vi "NanotecSMCPD.get parameters.vi"(0 "i ref in":refnum<vi>, 5 "error in (no error)":errorcluster) -> (7 "ReverseDirection?":bool[](array[boolean]), 8 "startFrequency [unit/s]":dbl[](array[numeric]), 9 "PhaseCurrent [A]":dbl[](array[numeric]), 11 "name":string[](array[string]), 12 "stopFrequency [unit/s]":dbl[](array[numeric]), 13 "unit":string[](array[string]), 14 "i ref out":refnum<vi>, 15 "acceleration [unit/s^2]":dbl[](array[numeric]), 16 "minRange [unit]":dbl[](array[numeric]), 17 "maxRange[unit]":dbl[](array[numeric]), 18 "scaling [unit]":dbl[](array[numeric]), 19 "error out":errorcluster)   [LabVIEW 2014, in "NanotecSMCPD.lvlib"]
doc: "Gets the parameters required for configuring the axes."
uses:
  NanotecSMCPD.lvlib
  CS_Core/BaseProcess/BaseProcess.lvlib
  CS_Core/CSSystem/CoreLib/CoreLib.lvlib
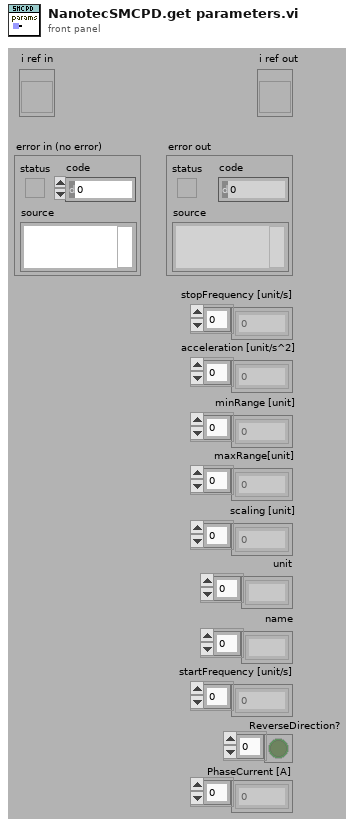
[diagram p1: front panel]
types:
  T1 = typedef "BaseProcess.lvlib/BaseProcess.i attribute.ctl" = cluster{"EventStatus":string, "EventError":i32, "PresetEvtWatchD":i32, "PresetPdcWatchD":i32, "EventTimeout":i32, "PeriodicInterval":i32, "Interface":string[], "Address":string[], "Special":string[], "PeriodicError":i32, "PeriodicStatus":string, "SuperProc":string, "Descriptors":T2[], "CaseRef":refnum<vi>, "PdcRef":refnum<vi>, "Thread Ref":refnum<vi>, "eventErrorID":i32, "eventStatusID":i32, "periodicErrorID":i32, "periodicStatusID":i32, "pdcCtrID":i32}
  T2 = typedef "BaseProcess.lvlib/BaseProcess.descriptor definition.ctl" = cluster{"selector":string, "descriptor":T3}
  T3 = typedef "BaseProcess.lvlib/BaseProcess.descriptor string definition.ctl" = string
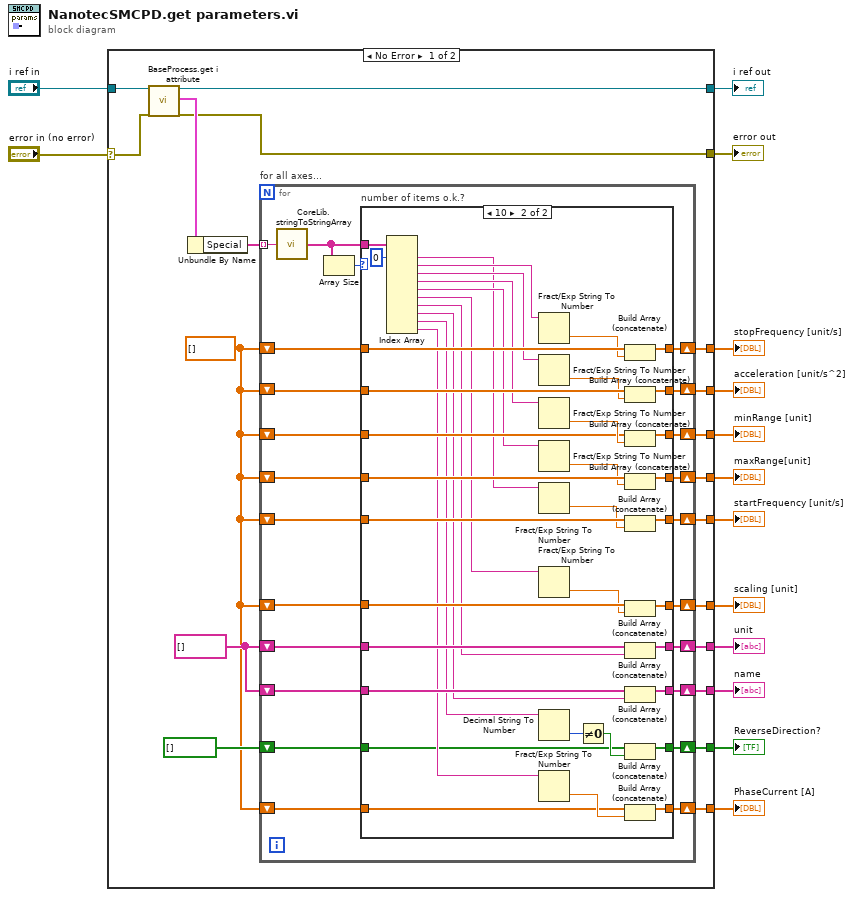
[diagram p0: block diagram]
diagram:
  n1 = case shown="No Error" "error in (no error)" {
    selector: "error in (no error)" -> [w29 w108]
    tunnel: "i ref in" -> [w33 w109]
    tunnel: [w31 w109] -> w13
    tunnel: [w30 w108] -> w12
    tunnel: [w27 _] -> w10
    tunnel: [w26 _] -> w9
    tunnel: [w25 _] -> w8
    tunnel: [w24 _] -> w7
    tunnel: [w23 _] -> w4
    tunnel: [w22 _] -> w6
    tunnel: [w21 _] -> w5
    tunnel: [w19 _] -> w3
    tunnel: [w16 _] -> w2
    tunnel: [w15 _] -> w1
    frame No Error {
      w20 = string[] []
      w17 = dbl[] []
      n2 = call "BaseProcess.get i attribute.vi"("i ref in"=w33, "error in (no error)"=w29) -> ("i ref out"=w31:refnum<vi>, "i attribute"=w32:T1, "error out"=w30:errorcluster)  [unwired: 15 in]
      n3 = Unbundle By Name(w32) -> ("Special"=w28:string[])
      n4 = for "for all axes..." {
        tunnel: w28 -> [w54] mode=indexing
        shift-right: [w55] -> w27
        shift-left: w17 -> [w56]
        shift-right: [w51] -> w26
        shift-left: w17 -> [w50]
        shift-right: [w49] -> w25
        shift-left: w17 -> [w48]
        shift-right: [w47] -> w24
        shift-left: w17 -> [w46]
        shift-right: [w44] -> w23
        shift-left: w17 -> [w45]
        shift-right: [w40] -> w22
        shift-left: w20 -> [w43]
        shift-right: [w41] -> w21
        shift-left: w20 -> [w42]
        shift-right: [w39] -> w19
        shift-left: w17 -> [w38]
        shift-right: [w35] -> w16
        shift-left: bool[] [] ("array") -> [w37]
        shift-right: [w34] -> w15
        shift-left: w17 -> [w36]
        n5 = call "CoreLib.stringToStringArray.vi"("String"=w54) -> ("Array"=w52:string[])
        n6 = Array Size(array=w52) -> (size(s)=w53:i32)
        n7 = case "number of items o.k.?" shown="10" w53 {
          tunnel: w56 -> [w66 w107]
          tunnel: [w66 w106] -> w55
          tunnel: w52 -> [_ w105]
          tunnel: [w65 w102] -> w51
          tunnel: w50 -> [w65 w101]
          tunnel: [w64 w99] -> w49
          tunnel: w48 -> [w64 w97]
          tunnel: [w63 w96] -> w47
          tunnel: w46 -> [w63 w95]
          tunnel: w45 -> [w62 w93]
          tunnel: [w62 w91] -> w44
          tunnel: w43 -> [w61 w90]
          tunnel: w42 -> [w60 w89]
          tunnel: [w60 w88] -> w41
          tunnel: [w61 w87] -> w40
          tunnel: [w59 w84] -> w39
          tunnel: w38 -> [w59 w86]
          tunnel: w37 -> [w58 w70]
          tunnel: w36 -> [w57 w69]
          tunnel: [w58 w68] -> w35
          tunnel: [w57 w67] -> w34
          frame 0, Default {
          }
          frame 10 {
            n8 = Index Array(array=w105, index #1=0 ("index")) -> (element #1=w79:string, element #2=w83:string, element #3=w82:string, element #4=w81:string, element #5=w80:string, element #6=w78:string, element #7=w77:string, element #8=w76:string, element #9=w75:string, element #10=w74:string)  [unwired: 9 in]
            n9 = Fract/Exp String To Number(string=w83) -> (number=w103:dbl)  [unwired: 3 in, 1 out]
            n10 = Fract/Exp String To Number(string=w82) -> (number=w100:dbl)  [unwired: 3 in, 1 out]
            n11 = Fract/Exp String To Number(string=w81) -> (number=w98:dbl)  [unwired: 3 in, 1 out]
            n12 = Fract/Exp String To Number(string=w80) -> (number=w94:dbl)  [unwired: 3 in, 1 out]
            n13 = Fract/Exp String To Number(string=w79) -> (number=w85:dbl)  [unwired: 3 in, 1 out]
            n14 = Fract/Exp String To Number(string=w78) -> (number=w92:dbl)  [unwired: 3 in, 1 out]
            n15 = Decimal String To Number(string=w75) -> (number=w72:i32)  [unwired: 2 in, 1 out]
            n16 = Fract/Exp String To Number(string=w74) -> (number=w73:dbl)  [unwired: 3 in, 1 out]
            n17 = Not Equal To 0?(x=w72) -> (x != 0?=w71:bool)
            n18 = Build Array (concatenate)(w107, w103) -> (w106:dbl[])
            n19 = Build Array (concatenate)(w101, w100) -> (w102:dbl[])
            n20 = Build Array (concatenate)(w97, w98) -> (w99:dbl[])
            n21 = Build Array (concatenate)(w95, w94) -> (w96:dbl[])
            n22 = Build Array (concatenate)(w86, w85) -> (w84:dbl[])
            n23 = Build Array (concatenate)(w93, w92) -> (w91:dbl[])
            n24 = Build Array (concatenate)(w90, w77) -> (w87:string[])
            n25 = Build Array (concatenate)(w89, w76) -> (w88:string[])
            n26 = Build Array (concatenate)(w70, w71) -> (w68:bool[])
            n27 = Build Array (concatenate)(w69, w73) -> (w67:dbl[])
          }
        }
      }
    }
    frame Error {
    }
  }
  "error out" <- w12
  "i ref out" <- w13
  "stopFrequency [unit/s]" <- w10
  "acceleration [unit/s^2]" <- w9
  "minRange [unit]" <- w8
  "maxRange[unit]" <- w7
  "scaling [unit]" <- w4
  "unit" <- w6
  "name" <- w5
  "startFrequency [unit/s]" <- w3
  "ReverseDirection?" <- w2
  "PhaseCurrent [A]" <- w1
